vi "Serial Open.vi"(8 "Error In":errorcluster, 10 "Baud Rate":u32=9600, 11 "LINX Device Config":T1) -> (0 "Error Out":errorcluster, 3 "LINX Device Config":T1)   [LabVIEW 2020, in "LMH-LINX.lvlib" / "Device.lvlib"]
doc: "Open the serial port associated with the LINX device."
uses:
  Device.lvlib
  Type Defs/LINX Device Config.ctl
  Type Defs/Interface.ctl
  Type Defs/TCP Config.ctl
  Type Defs/Channels.ctl
  Type Defs/Error Type.ctl
  <vilib>/Instr/_visa.llb/VISA Configure Serial Port (Instr).vi
  LMH-LINX.lvlib
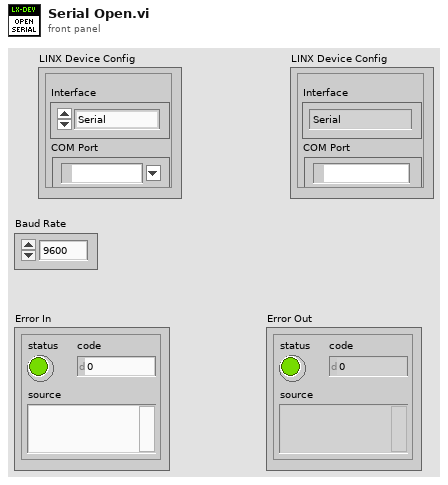
[diagram p1: front panel]
types:
  T1 = typedef "LMH-LINX.lvlib/Device.lvlib/LINX Device Config.ctl" = cluster{"Interface":T2, "COM Port":refnum<visa-resource-name>, "TCP Configuration":T3, "Device Family":u8, "Device ID":u8, "Device Name":string, "TCP Ref":refnum<k5>, "Channels":T4}
  T2 = typedef "LMH-LINX.lvlib/Interface.ctl" = enum16{"Serial", "TCP"}
  T3 = typedef "LMH-LINX.lvlib/Device.lvlib/TCP Config.ctl" = cluster{"IP Address":string, "Port":u16}
  T4 = typedef "LMH-LINX.lvlib/Channels.ctl" = cluster{"DI":u8[], "DO":u8[], "AI":u8[], "AO":u8[], "PWM":u8[], "QE":u8[], "UART":u8[], "I2C 2":u8[], "SPI":u8[], "CAN":u8[], "Servo":u8[], "AI Ref (V)":dbl, "AI Resolution (Bits)":u8, "AO Ref (V)":dbl, "AO Resolution (Bits)":u8}
  T5 = typedef "LMH-LINX.lvlib/Error Type.ctl" = enum16{"Unknown", "Timeout", "Corrupt Return Packet", "Unable To Connect", "Command Not Supported", "Channel DNE", "Invalid COM Config", "Firmware Version Mismatch", "myRIO Support", "CMD Specific Error", "Local IO Not Supported"}
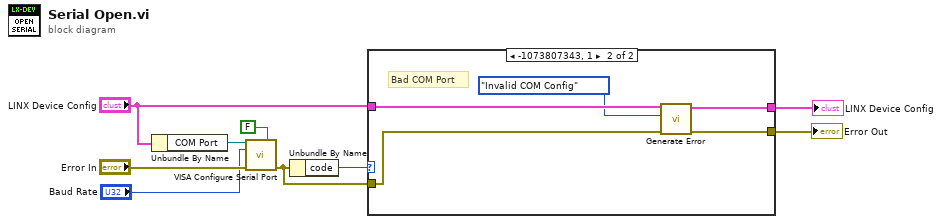
[diagram p0: block diagram]
diagram:
  n1 = Unbundle By Name("LINX Device Config") -> ("COM Port"=w9:refnum<visa-resource-name>)
  n2 = call-poly "VISA Configure Serial Port"("VISA resource name"=w9, "Enable Termination\nChar (T)"=FALSE ("Enable Termination\nChar (T)"), "baud rate (9600)"="Baud Rate", "error in (no error)"="Error In") -> ("error out"=w4:errorcluster)  [unwired: 10 in, 1 out]
  n3 = Unbundle By Name(w4) -> ("code"=w5:i32)
  n4 = case shown="-1073807343, 1" w5 {
    tunnel: w4 -> [w10 w13]
    tunnel: "LINX Device Config" -> [w11 w16]
    tunnel: [w11 w15] -> w2
    tunnel: [w10 w14] -> w1
    frame 0, Default {
    }
    frame -1073807343, 1 {
      # "Bad COM Port"
      n5 = call "Generate Error.vi"("Error In"=w13, "Error Type"=Error_Type."Invalid COM Config", "LINX Device Config"=w16) -> ("Error Out"=w14:errorcluster, "Dup LINX Device Config"=w15:T1)  [unwired: 7 in]
    }
  }
  "Error Out" <- w1
  "LINX Device Config" <- w2
